vi "UV-VIS Init Param.vi"(7 "error in (no error)":errorcluster, 10 "UV-VIS detector in":refnum<class "CCD_camera.lvclass">) -> (0 "error out":errorcluster, 3 "UV-VIS detector out":refnum<class "CCD_camera.lvclass">)   [LabVIEW 2020, in "CCD_camera.lvclass"]
uses:
  CCD_camera.lvclass
  dependecies/AcquisitionMode_mode typedef.ctl
  methods/atmcd32d.llb/ReadMode_mode typedef.ctl
  methods/atmcd32d.llb/HSSpeed_type typedef.ctl
  methods/atmcd32d.llb/TriggerMode_mode typedef.ctl
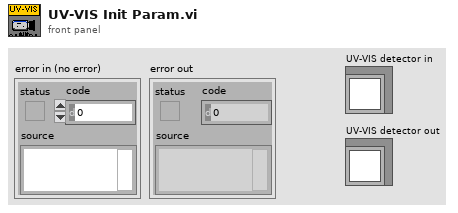
[diagram p1: front panel]
types:
  T1 = typedef "TriggerMode_mode typedef.ctl" = enum16{"Internal", "External", "N/A (2)", "N/A (3)", "N/A (4)", "N/A (5)", "External Start", "External Exposure (Bulb)", "N/A (8)", "External FVB EM", "Software", "N/A (11)", "External Charge Shifting"}
  T2 = typedef "ReadMode_mode typedef.ctl" = enum16{"Full Vertical Binning", "Multi-Track", "Random-Track", "Single-Track", "Image"}
  T3 = typedef "AcquisitionMode_mode typedef.ctl" = enum16{"Reserved (0)", "Single Scan", "Accumulate", "Kinetics", "Fast Kinetics", "Run Till Abort for non-Frame Transfer", "Frame Transfer", "Run Till Abort for Frame Transfer", "Reserved (8)", "Time Delayed Integration"}
  T4 = typedef "HSSpeed_type typedef.ctl" = enum16{"EM Amp", "Conventional Amp"}
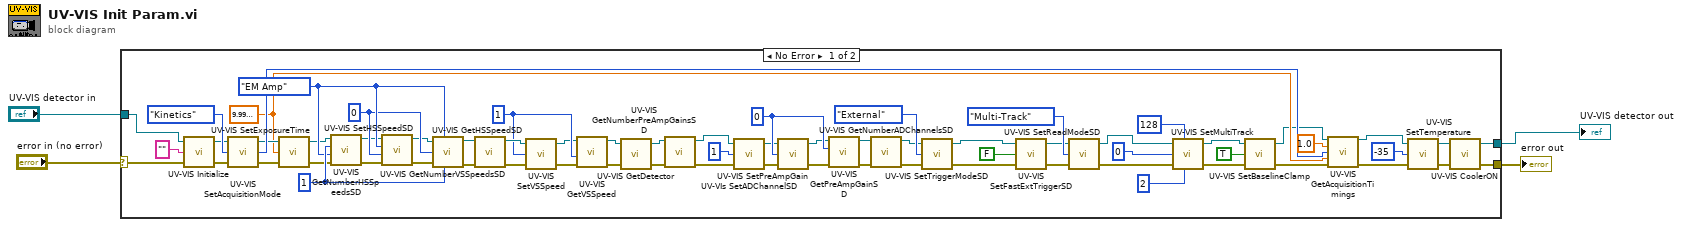
[diagram p0: block diagram]
diagram:
  n1 = case shown="No Error" "error in (no error)" {
    selector: "error in (no error)" -> [w35 w73]
    tunnel: [w8 w73] -> w4
    tunnel: [w6 w72] -> w2
    tunnel: "UV-VIS detector in" -> [w34 w72]
    frame No Error {
      w49 = HSSpeed_type_typedef."EM Amp" ("type")
      w41 = 0 ("index HSSpeed")
      w23 = 1 ("index VSSpeed")
      w58 = 0 ("index preamp gain")
      w28 = sgl 0.0001 ("time")
      w64 = 1 ("channel HSSpeed")
      n2 = call "UV-VIS Initialize.vi"("error in (no error)"=w35, "directory (\"\")"="" ("directory (\"\")"), "UV-VIS in"=w34) -> ("error out"=w39:errorcluster, "Control out"=w33:refnum<class "CCD_camera.lvclass">)  [unwired: 1 out]
      n3 = call "UV-VIS SetAcquisitionMode.vi"("error in (no error)"=w39, "mode"=AcquisitionMode_mode_typedef."Kinetics", "Control in"=w33) -> ("error out"=w44:errorcluster, "DLL error code"=w45:u32, "Control out"=w32:refnum<class "CCD_camera.lvclass">)
      n4 = call "UV-VIS SetExposureTime.vi"("error in (no error)"=w44, "time"=w28, "Control in"=w32) -> ("error out"=w56:errorcluster, "Control out"=w31:refnum<class "CCD_camera.lvclass">)  [unwired: 1 out]
      n5 = call "UV-VIS GetNumberHSSpeedsSD.vi"("error in (no error)"=w56, "type"=w49, "channel"=w64, "Control in"=w31) -> ("error out"=w65:errorcluster, "Control out"=w30:refnum<class "CCD_camera.lvclass">)  [unwired: 2 out]
      n6 = call "UV-VIS SetHSSpeedSD.vi"("error in (no error)"=w65, "index"=w41, "type"=w49, "Control in"=w30) -> ("error out"=w66:errorcluster, "Control out"=w29:refnum<class "CCD_camera.lvclass">)  [unwired: 1 in, 1 out]
      n7 = call "UV-VIS GetHSSpeedSD.vi"("Control in"=w29, "type"=w49, "index"=w41, "error in (no error)"=w66, "channel"=w64) -> ("Control out"=w26:refnum<class "CCD_camera.lvclass">, "error out"=w55:errorcluster)  [unwired: 2 out]
      n8 = call "UV-VIS GetNumberVSSpeedsSD.vi"("error in (no error)"=w55, "Control in"=w26) -> ("error out"=w63:errorcluster, "Control out"=w24:refnum<class "CCD_camera.lvclass">)  [unwired: 2 in, 2 out]
      n9 = call "UV-VIS SetVSSpeed.vi"("error in (no error)"=w63, "index"=w23, "Control in"=w24) -> ("error out"=w62:errorcluster, "Control out"=w22:refnum<class "CCD_camera.lvclass">)  [unwired: 1 out]
      n10 = call "UV-VIS GetVSSpeed.vi"("error in (no error)"=w62, "index"=w23, "Control in"=w22) -> ("error out"=w54:errorcluster, "Control out"=w20:refnum<class "CCD_camera.lvclass">)  [unwired: 1 in, 2 out]
      n11 = call "UV-VIS GetDetector.vi"("UV-VIS in"=w20, "error in (no error)"=w54) -> ("UV-VIS out"=w19:refnum<class "CCD_camera.lvclass">, "error out"=w53:errorcluster)  [unwired: 3 in, 3 out]
      n12 = call "UV-VIS GetNumberPreAmpGainsSD.vi"("error in (no error)"=w53, "UV-VIS in"=w19) -> ("error out"=w43:errorcluster, "UV-VIS out"=w18:refnum<class "CCD_camera.lvclass">)  [unwired: 2 in, 2 out]
      n13 = call "UV-VIs SetADChannelSD.vi"("error in (no error)"=w43, "channel"=1, "Control in"=w18) -> ("error out"=w42:errorcluster, "Control out"=w21:refnum<class "CCD_camera.lvclass">)  [unwired: 1 out]
      n14 = call "UV-VIS SetPreAmpGain.vi"("error in (no error)"=w42, "index"=w58, "Control in"=w21) -> ("error out"=w68:errorcluster, "Control out"=w16:refnum<class "CCD_camera.lvclass">)  [unwired: 1 out]
      n15 = call "UV-VIS GetPreAmpGainSD.vi"("error in (no error)"=w68, "index"=w58, "Control in"=w16) -> ("error out"=w48:errorcluster, "Control out"=w15:refnum<class "CCD_camera.lvclass">)  [unwired: 1 in, 2 out]
      n16 = call "UV-VIS GetNumberADChannelsSD.vi"("error in (no error)"=w48, "Control in"=w15) -> ("error out"=w52:errorcluster, "Control out"=w13:refnum<class "CCD_camera.lvclass">)  [unwired: 2 in, 2 out]
      n17 = call "UV-VIS SetTriggerModeSD.vi"("error in (no error)"=w52, "mode"=TriggerMode_mode_typedef."External", "Control in"=w13) -> ("error out"=w71:errorcluster, "Control out"=w12:refnum<class "CCD_camera.lvclass">)  [unwired: 1 out]
      n18 = call "UV-VIS SetFastExtTriggerSD.vi"("error in (no error)"=w71, "mode"=FALSE ("Fast external mode"), "Control in"=w12) -> ("error out"=w51:errorcluster, "Control out"=w14:refnum<class "CCD_camera.lvclass">)  [unwired: 1 out]
      n19 = call "UV-VIS SetReadModeSD.vi"("error in (no error)"=w51, "mode"=ReadMode_mode_typedef."Multi-Track" ("readout  mode"), "Control in"=w14) -> ("error out"=w67:errorcluster, "Control out"=w17:refnum<class "CCD_camera.lvclass">)  [unwired: 1 out]
      n20 = call "UV-VIS SetMultiTrack.vi"("Control in"=w17, "height"=128, "offset"=0, "error in (no error)"=w67, "number"=2) -> ("Control out"=w25:refnum<class "CCD_camera.lvclass">, "error out"=w37:errorcluster)  [unwired: 3 out]
      n21 = call "UV-VIS SetBaselineClamp.vi"("error in (no error)"=w37, "state"=TRUE ("Base line Clamp"), "Control in"=w25) -> ("error out"=w36:errorcluster, "Control out"=w27:refnum<class "CCD_camera.lvclass">)  [unwired: 1 out]
      n22 = call "UV-VIS GetAcquisitionTimings.vi"("Control in"=w27, "accumulate input"=sgl 1.0, "kinetic input"=w45, "exposure input"=w28, "error in (no error)"=w36) -> ("Control out"=w11:refnum<class "CCD_camera.lvclass">, "error out"=w10:errorcluster)  [unwired: 5 in, 4 out]
      n23 = call "UV-VIS SetTemperature.vi"("error in (no error)"=w10, "temperature"=-35, "UV-VIS detector in"=w11) -> ("error out"=w9:errorcluster, "UV-VIS detector out"=w7:refnum<class "CCD_camera.lvclass">)  [unwired: 1 out]
      n24 = call "UV-VIS CoolerON.vi"("error in (no error)"=w9, "UV-VIS  in"=w7) -> ("error out"=w8:errorcluster, "UV-VIS  out"=w6:refnum<class "CCD_camera.lvclass">)  [unwired: 1 in, 1 out]
    }
    frame Error {
    }
  }
  "UV-VIS detector out" <- w2
  "error out" <- w4
